vi "Import config from file.vi"(8 "error in (no error)":errorcluster, 11 "Node Ptr":u64 format="%.0x") -> (0 "error out":errorcluster)   [LabVIEW 2017, in "Shared Variables CD 2.0 Configuration.lvlib"]
uses:
  Shared Variables CD 2.0 Configuration.lvlib
  Public/Documents/National Instruments/NI VeriStand 2017/Custom Devices/Shared Variables CD 2.0/data/ImportExport.lvlibp/Operation.ctl
  Shared/SV Global.vi
  Public/Documents/National Instruments/NI VeriStand 2017/Custom Devices/Shared Variables CD 2.0/data/ImportExport.lvlibp
  <vilib>/NI VeriStand/Custom Device API/Custom Device API.lvlib
  Support/ChannelVS/ChannelVS.lvclass
panel:
  in  "Tag":string
  # "Wait...."
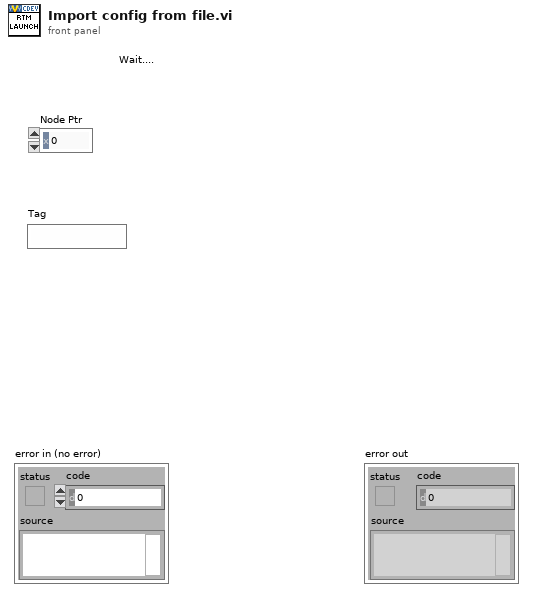
[diagram p1: front panel]
types:
  T1 = typedef "ImportExport.lvlibp/Operation.ctl" = enum16{"Import", "Export"}
  T2 = typedef "Custom Device API.lvlib/Custom Device Item Ref.ctl" = u64
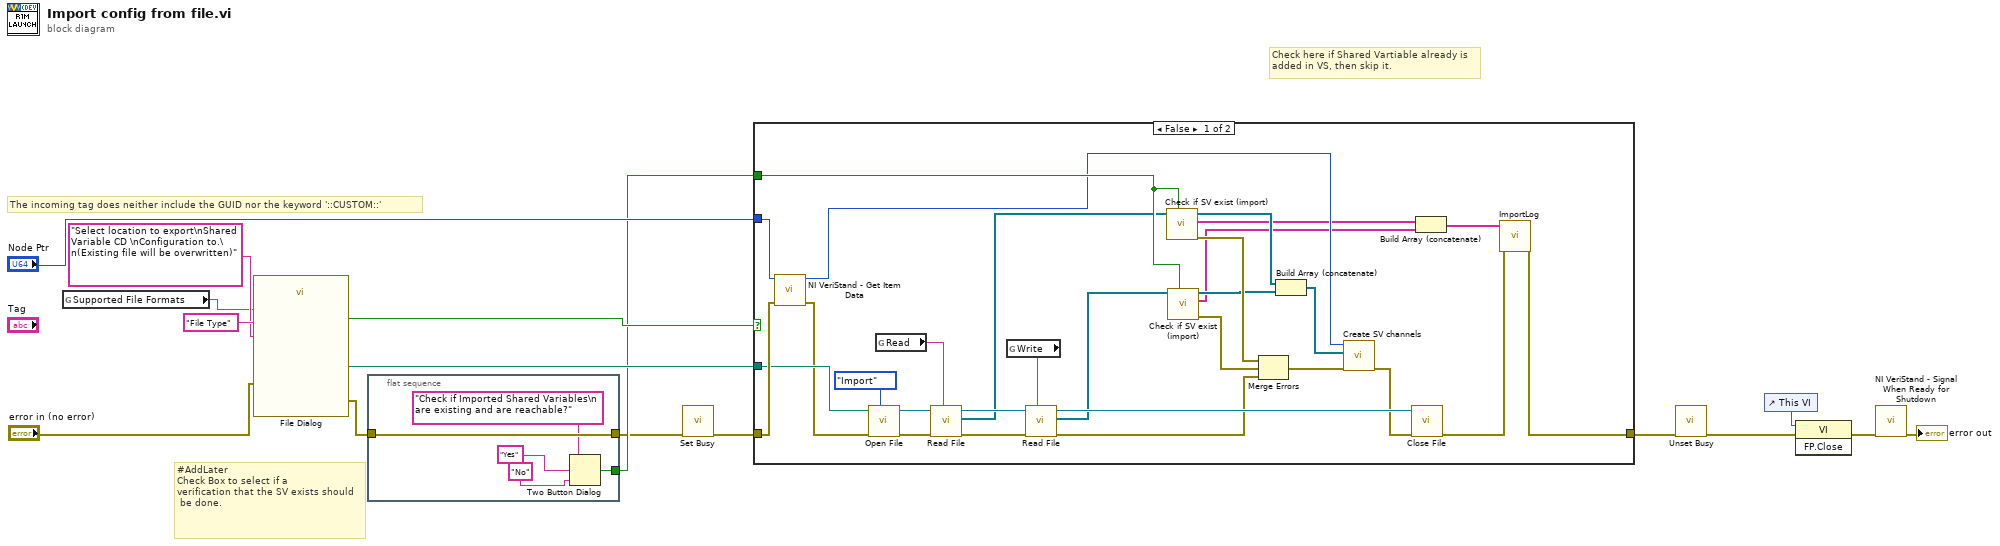
[diagram p0: block diagram]
diagram:
  # "Check here if Shared Vartiable already is\nadded in VS, then skip it."
  # "#AddLater\nCheck Box to select if a\nverification that the SV exists should\n be done."
  # "The incoming tag does neither include the GUID nor the keyword '::CUSTOM::'"
  n1 = global read "SV Global.vi" "Supported File Formats"() -> (w7:string)
  n2 = call "File Dialog"("prompt"="Select location to export\nShared Variable CD \nConfiguration to.\n(Existing file will be overwritten)", "error in"="error in (no error)", "pattern (all files)"=w7, "pattern label"="File Type") -> ("selected path"=w12:path, "cancelled"=w13:bool, "error out"=w6:errorcluster)  [unwired: 8 in, 1 out]
  n3 = flat-sequence {
    tunnel: [w21] -> w4
    tunnel: w6 -> [w21]
    tunnel: [w17] -> w5
    frame #0 {
      n4 = Two Button Dialog(message="Check if Imported Shared Variables\n are existing and are reachable?", 1:"No" ("F button name (\"Cancel\")"), 2:"Yes" ("T button name (\"OK\")")) -> (T button?=w17:bool)
    }
  }
  n5 = call <vilib>:"Set Busy.vi"("error in (no error)"=w4) -> ("error out"=w3:errorcluster)  [unwired: 9 in, 1 out]
  n6 = case shown="False" w13 {
    tunnel: [w25 w51] -> w2
    tunnel: w3 -> [w49 w51]
    tunnel: w12 -> [w48 _]
    tunnel: "Node Ptr" -> [w41 _]
    tunnel: w5 -> [w38 _]
    frame False {
      n7 = call <vilib>:"NI VeriStand - Get Item Data.vi"("error in (no error)"=w49, "Item Ref in"=w41) -> ("error out"=w32:errorcluster, "Item Ref out"=w37:T2)  [unwired: 6 in, 2 out]
      n8 = call "Open File.vi"("Operation"=Operation."Import", "error in (no error)"=w32, "Path"=w48) -> ("error out"=w42:errorcluster, "ConfigFile out"=w47:refnum<class "ConfigFile.lvclass">)  [unwired: 7 in]
      n9 = global read "SV Global.vi" "Read"() -> (w35:string)
      n10 = call "Read File.vi"("Channel Direction"=w35, "error in (no error)"=w42, "ConfigFile in"=w47) -> ("error out"=w45:errorcluster, "Channels"=w30:refnum<class "Channel.lvclass">[], "ConfigFile out"=w46:refnum<class "ConfigFile.lvclass">)  [unwired: 6 in]
      n11 = global read "SV Global.vi" "Write"() -> (w36:string)
      n12 = call "Read File.vi"("Channel Direction"=w36, "error in (no error)"=w45, "ConfigFile in"=w46) -> ("error out"=w43:errorcluster, "Channels"=w31:refnum<class "Channel.lvclass">[], "ConfigFile out"=w44:refnum<class "ConfigFile.lvclass">)  [unwired: 6 in]
      n13 = call "Check if SV exist (import).vi"("Check if SV Exists?"=w38, "Channels in"=w30) -> ("error out"=w39:errorcluster, "Missing Variables"=w24:string[], "Channels in 2"=w29:refnum<class "Channel.lvclass">[])  [unwired: 7 in]
      n14 = call "Check if SV exist (import).vi"("Check if SV Exists?"=w38, "Channels in"=w31) -> ("error out"=w40:errorcluster, "Missing Variables"=w23:string[], "Channels in 2"=w28:refnum<class "Channel.lvclass">[])  [unwired: 7 in]
      n15 = Merge Errors(w39, w40, w43) -> (w34:errorcluster)
      n16 = Build Array (concatenate)(w29, w28) -> (w27:refnum<class "Channel.lvclass">[])
      n17 = call "Create SV channels.vi"("error in"=w34, "Variable List"=w27, "Custom Device in"=w37) -> ("error out"=w33:errorcluster)  [unwired: 7 in, 1 out]
      n18 = call "Close File.vi"("error in (no error)"=w33, "ConfigFile in"=w44) -> ("error out"=w26:errorcluster)  [unwired: 9 in]
      n19 = Build Array (concatenate)(w24, w23) -> (w22:string[])
      n20 = call "ImportLog.vi"("error in (no error)"=w26, "Missing Variables"=w22) -> ("error out"=w25:errorcluster)  [unwired: 9 in]
    }
    frame True {
    }
  }
  n21 = call <vilib>:"Unset Busy.vi"("error in (no error)"=w2) -> ("error out"=w1:errorcluster)  [unwired: 10 in]
  n22 = control-ref of="This VI"() -> (w10:refnum<vi>)
  n23 = invoke class="VI" method="FP.Close"(reference=w10, error in=w1) -> (error out=w11:errorcluster)  [unwired: 1 in, 2 out]
  n24 = call <vilib>:"NI VeriStand - Signal When Ready for Shutdown.vi"("error in (no error)"=w11) -> ("error out"=→"error out":errorcluster)  [unwired: 10 in]
